vi "add to sim log.vi"(8 "error in (no error)":errorcluster, 11 "log":string) -> (0 "error out":errorcluster)   [LabVIEW 2019, in "libSimulationControl.lvlib"]
doc: "void add_to_sim_log(const char* log);"
uses:
  libSimulationControl.lvlib
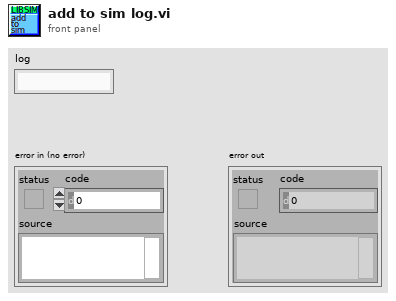
[diagram p1: front panel]
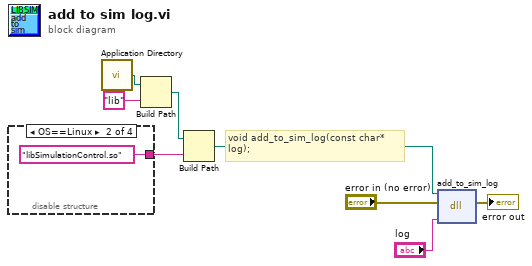
[diagram p0: block diagram]
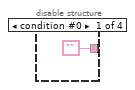
[diagram p2: hidden frame]
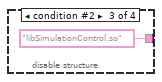
[diagram p3: hidden frame]
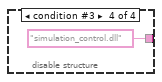
[diagram p4: hidden frame]
diagram:
  # "void add_to_sim_log(const char* log);"
  n1 = disable-structure shown="OS==Linux" {
    disable-tunnel: ["" "libSimulationControl.so" ("name or relative path") "libSimulationControl.so" ("name or relative path") "simulation_control.dll" ("name or relative path")] -> w2
    frame condition #0 {
    }
    frame condition #1 (active) {
    }
    frame condition #2 {
    }
    frame condition #3 {
    }
  }
  n2 = call <vilib>:"Application Directory.vi"() -> ("Application Directory"=w5:path)
  n3 = Build Path(base path=w5, name or relative path="lib") -> (appended path=w3:path)
  n4 = Build Path(base path=w3, name or relative path=w2) -> (appended path=w1:path)
  n5 = dll-call lib="home/paul/Schreibtisch/Biogas_plant_setup/LabView/lib/libSimulationControl/libSimulationControl.*" fn="add_to_sim_log"(path in=w1, error in="error in (no error)", "log"="log") -> (error out=→"error out":errorcluster)  [unwired: 3 in, 1 out]
